vi "Increasing_File_Name.vi"(1 "Base AVI  path":path) -> (0 "Final AVI path":path)   [LabVIEW 2010]
panel:
  in  "Saved path":path
  in  "id":u32
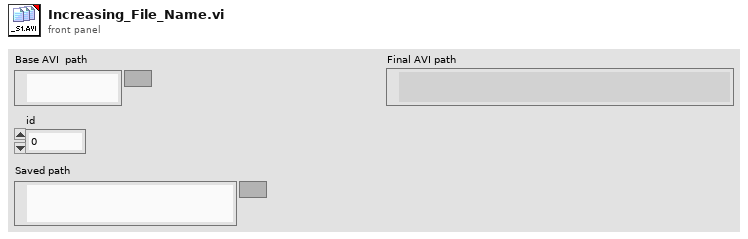
[diagram p1: front panel]
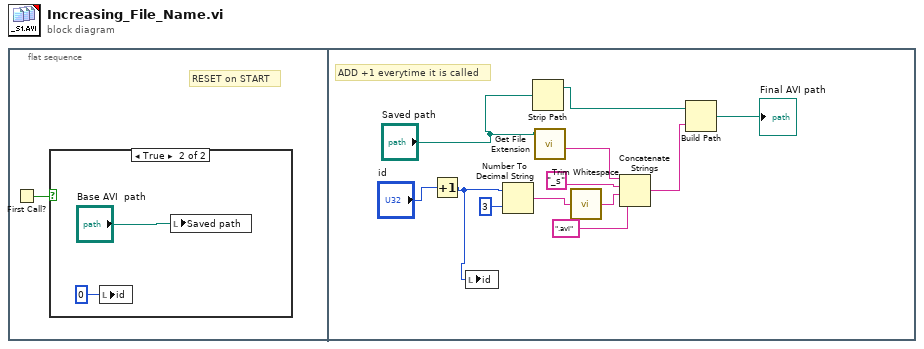
[diagram p0: block diagram]
diagram:
  n1 = flat-sequence {
    frame #0 {
      # "RESET on START"
      n2 = First Call?() -> (First Call?: T/F=w1:bool)
      n3 = case shown="True" w1 {
        frame False {
        }
        frame True {
          n4 = local write "id"(u32 0 ("id")) -> ()
          n5 = local write "Saved path"("Base AVI  path") -> ()
        }
      }
    }
    frame #1 {
      # "ADD +1 everytime it is called"
      n6 = Increment(x="id") -> (x+1=w5:u32)
      n7 = local write "id"(w5) -> ()
      n8 = Number To Decimal String(number=w5, width (-)=i16 3) -> (decimal integer string=w10:string)
      n9 = Strip Path(path="Saved path") -> (stripped path=w15:path)  [unwired: 1 out]
      n10 = call <vilib>:"Get File Extension.vi"("file"="Saved path") -> ("filename without extension"=w13:string)  [unwired: 7 in, 3 out]
      n11 = call <vilib>:"Trim Whitespace.vi"("string"=w10) -> ("trimmed string"=w11:string)  [unwired: 1 in]
      n12 = Concatenate Strings(w13, "_s", w11, ".avi" ("string")) -> (w7:string)
      n13 = Build Path(base path=w15, name or relative path=w7) -> (appended path=→"Final AVI path":path)
    }
  }
